vi "te_readVal.vi"(0 "VISA In":refnum<visa-resource-name>, 5 "Hex Address":string="00", 7 "Command":string="01", 11 "Error In":errorcluster) -> (4 "VISA Out":refnum<visa-resource-name>, 6 "Response Dec":dbl, 8 "Response":dbl, 10 "Response Hex":string, 15 "error out":errorcluster)   [LabVIEW 2018]
doc: "The Basic Serial Read and Write example performs a Serial Port Read, a Serial Port Write, or a combination of these actions. The user selects the actions (read or write) on the front panel. If both are selected, the VI will write the data first, read data, and then close the VISA session that is opened to the port. This VI will wait until the specified number of bytes is received at the port. Only the number of bytes specified will be read.\n\nINSTRUCTIONS:\n1) Select the serial resource and configuration parameters (baud rate, data bits, parity, stop bits, flow control).\n2) Select the operations to be performed. \n3) Connect the serial port to your device. If no device is available, perform a loopback test by doing one of the following. Short pins 2 and 3 on a RS-232 cable or short pin 4 to pin 8 and pin 5 to pin 9 on a RS-485/422 cable. \n4) Run the VI to see the data read. (The \"read string\" will match the \"string to write\" if a loopback test was performed.)\n\nNote: The parameters set for the serial port must match the parameters of the connected instrument or device. In this example, the bytes to read parameter specifies the number of bytes that the serial port reads. If there were more bytes at the port than the number specified in bytes to read, those bytes would not be read. Also, if you specify to read more bytes than the number of bytes actually read, you might receive a timeout error message.\n\nOn the block diagram, the Configure Serial Port VI sets the configuration parameters. The front panel displays the controls used to configure the basic parameters, such as baud rate, data bits, and parity. Constants configure the other parameters the user probably does not need set. After the VISA Configure Serial Port VI opens the VISA session and configures the port, the VI passes the VISA resource name to other VIs that perform operations on that VISA resource. The VISA Write function sends a command to the serial device and the VISA Read function returns data based on the command. The VISA Close function then closes the reference to the serial device. It is important to close the reference; otherwise communication through with that port through protocols other than VISA might not be possible."
panel:
  out "ByteCount":i32
  in  "Data":string
  out "Checksum":string
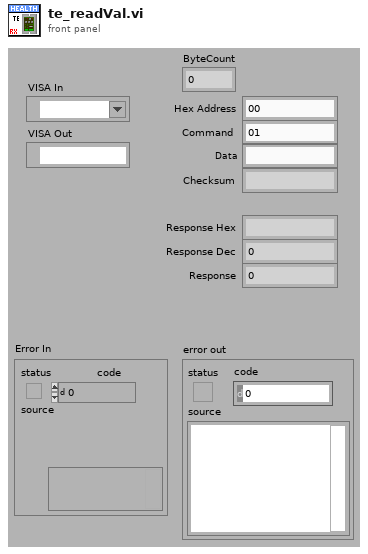
[diagram p1: front panel]
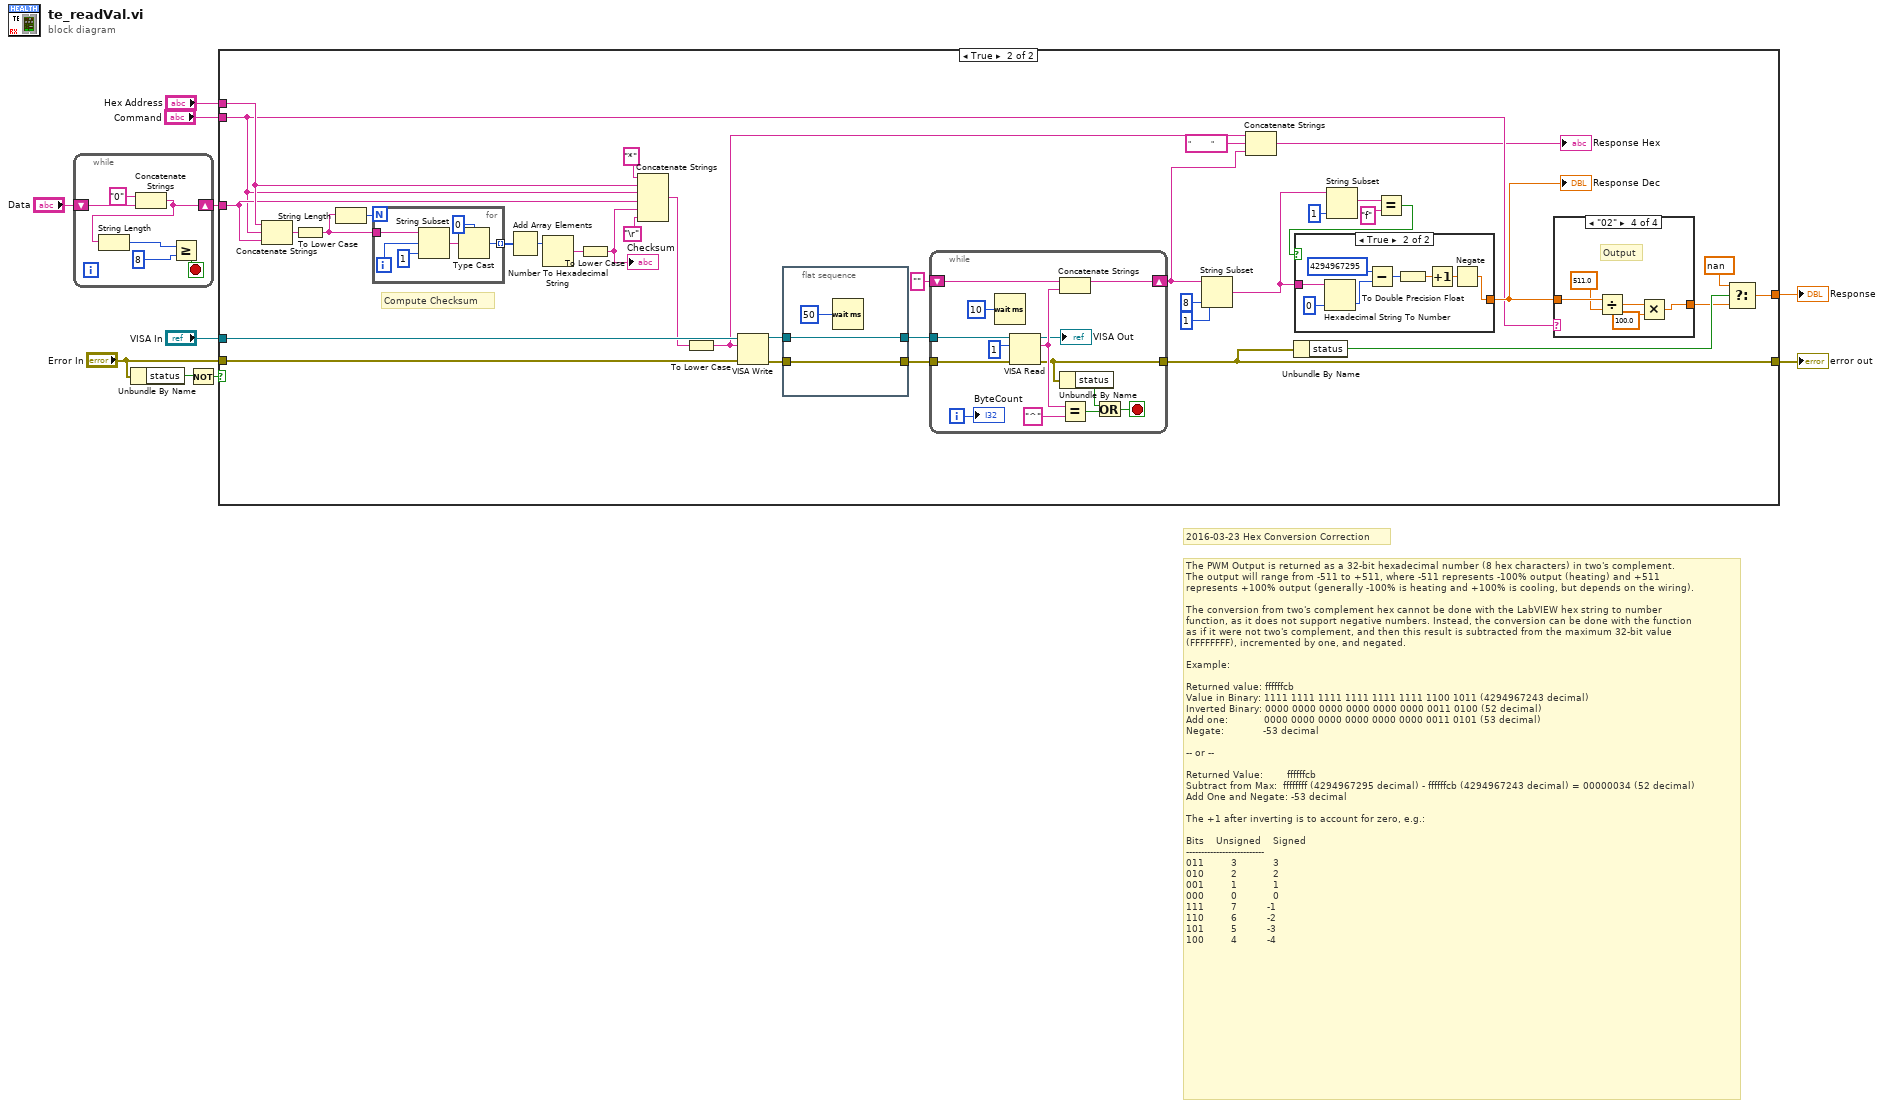
[diagram p0: block diagram]
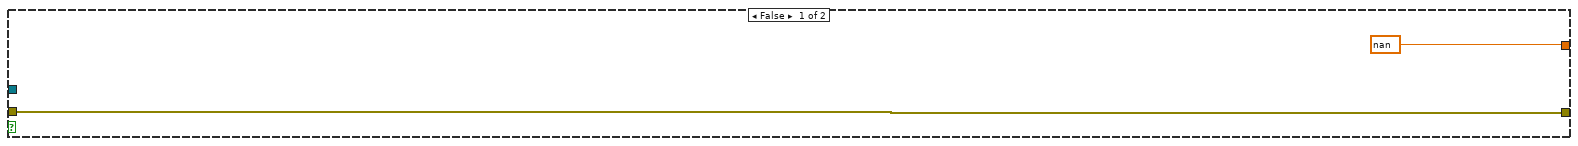
[diagram p2: hidden frame]
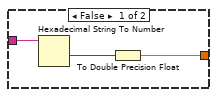
[diagram p3: hidden frame]
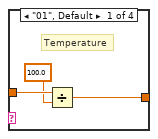
[diagram p4: hidden frame]
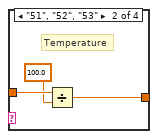
[diagram p5: hidden frame]
diagram:
  # "2016-03-23 Hex Conversion Correction"
  # "The PWM Output is returned as a 32-bit hexadecimal number (8 hex characters) in two's complement.\nThe output will range from -511 to +511, where -511 represents -100% output (heating) and +511\nrepresents +100% output (generally -100% is heating and +100% is cooling, but depends on the wiring).\n\nThe conversion from two's complement hex cannot be done with the LabVIEW hex string to number\nfunction, as it does not support negative numbers. Instead, the conversion can be done with the function\nas if it were not two's complement, and then this result is subtracted from the maximum 32-bit value\n(FFFFFFFF), incremented by one, and negated.\n\nExample:\n\nReturned value: ffffffcb\nValue in Binary: 1111 1111 1111 1111 1111 1111 1100 1011 (4294967243 decimal)\nInverted Binary: 0000 0000 0000 0000 0000 0000 0011 0100 (52 decimal)\nAdd one:            0000 0000 0000 0000 0000 0000 0011 0101 (53 decimal)\nNegate:             -53 decimal\n\n-- or --\n\nReturned Value:        ffffffcb\nSubtract from Max:  ffffffff (4294967295 decimal) - ffffffcb (4294967243 decimal) = 00000034 (52 decimal)\nAdd One and Negate: -53 decimal                \n\nThe +1 after inverting is to account for zero, e.g.:\n\nBits    Unsigned    Signed\n--------------------------\n011         3            3\n010         2            2\n001         1            1\n000         0            0\n111         7          -1\n110         6          -2\n101         5          -3\n100         4          -4"
  n1 = while {
    shift-right: [w14] -> w7
    shift-left: "Data" -> [w16]
    stop <- w11 stop-if-true
    n2 = Concatenate Strings("0" ("string"), w16) -> (w14:string)
    n3 = String Length(string=w14) -> (length=w12:i32)
    n4 = Greater Or Equal?(x=w12, y=8) -> (x >= y?=w11:bool)
  }
  n5 = Unbundle By Name("Error In") -> ("status"=w9:bool)
  n6 = Not(x=w9) -> (.not. x?=w10:bool)
  n7 = case shown="True" w10 {
    tunnel: "VISA In" -> [_ w54]
    tunnel: "Error In" -> [w18 w53]
    tunnel: [w18 w51] -> w8
    tunnel: w7 -> [_ w37]
    tunnel: [nan ("t") w39] -> w6
    tunnel: "Hex Address" -> [_ w38]
    tunnel: "Command" -> [_ w21]
    frame False {
    }
    frame True {
      # "Compute Checksum"
      n8 = Concatenate Strings(w38, w21, w37) -> (w43:string)
      n9 = To Lower Case(string=w43) -> (all lower case string=w45:string)
      n10 = String Length(string=w45) -> (length=w48:i32)
      n11 = for {
        N: w48 -> [_]
        tunnel: w45 -> [w63]
        tunnel: [w59] -> w47 mode=indexing
        i -> [w62]
        n12 = String Subset(string=w63, offset (0)=w62, length (rest)=1 ("length (rest)")) -> (substring=w60:string)
        n13 = Type Cast(type=u8 0, x=w60) -> (*(type *) &x=w59:u8)
      }
      n14 = Add Array Elements(numeric array=w47) -> (sum=w46:u8)
      n15 = Number To Hexadecimal String(2:w46) -> (0:w44:string)  [unwired: 1 in]
      n16 = To Lower Case(string=w44) -> (all lower case string=w42:string)
      "Checksum" <- w42
      n17 = Concatenate Strings("*", w38, w21, w37, w42, "\r") -> (w29:string)
      n18 = To Lower Case(string=w29) -> (all lower case string=w22:string)
      n19 = VISA Write(VISA resource name=w54, write buffer=w22, error in (no error)=w53) -> (VISA resource name out=w27:refnum<visa-resource-name>, error out=w28:errorcluster)  [unwired: 1 out]
      n20 = flat-sequence {
        tunnel: [w57] -> w25
        tunnel: w28 -> [w57]
        tunnel: [w56] -> w26
        tunnel: w27 -> [w56]
        frame #0 {
          n21 = Wait (ms)(milliseconds to wait=u32 50) -> ()  [unwired: 1 out]
        }
      }
      n22 = while {
        tunnel: [w69] -> w51
        tunnel: w26 -> [w71]
        tunnel: w25 -> [w77]
        shift-right: [w75] -> w23
        shift-left: "" ("read buffer") -> [w76]
        i -> [w66]
        stop <- w72 stop-if-true
        n23 = Wait (ms)(milliseconds to wait=u32 10) -> ()  [unwired: 1 out]
        n24 = VISA Read(VISA resource name=w71, byte count=u32 1, error in (no error)=w77) -> (VISA resource name out=→"VISA Out":refnum<visa-resource-name>, read buffer=w74:string, error out=w69:errorcluster)  [unwired: 1 out]
        n25 = Concatenate Strings(w76, w74) -> (w75:string)
        n26 = Unbundle By Name(w69) -> ("status"=w70:bool)
        n27 = Equal?(x=w74, y="^") -> (x = y?=w68:bool)
        n28 = Or(x=w70, y=w68) -> (x .or. y?=w72:bool)
        "ByteCount" <- w66
      }
      n29 = String Subset(string=w23, offset (0)=1, length (rest)=8 ("length (rest)")) -> (substring=w20:string)
      n30 = Concatenate Strings(w22, "          " ("string"), w23) -> (→"Response Hex":string)
      n31 = Unbundle By Name(w51) -> ("status"=w52:bool)
      n32 = String Subset(string=w20, length (rest)=1 ("length (rest)")) -> (substring=w31:string)  [unwired: 1 in]
      n33 = Equal?(x=w31, y="f") -> (x = y?=w33:bool)
      n34 = case shown="True" w33 {
        tunnel: [w80 w84] -> w40
        tunnel: w20 -> [w81 w88]
        frame False {
          n35 = Hexadecimal String To Number(string=w81) -> (number=w79:u32)  [unwired: 2 in, 1 out]
          n36 = To Double Precision Float(number=w79) -> (double precision float=w80:dbl)
        }
        frame True {
          n37 = Hexadecimal String To Number(string=w88, default (0uL)=u32 0 ("default (0 U32)")) -> (number=w86:u32)  [unwired: 1 in, 1 out]
          n38 = Subtract(x=u32 4294967295, y=w86) -> (x-y=w85:u32)
          n39 = To Double Precision Float(number=w85) -> (double precision float=w83:dbl)
          n40 = Increment(x=w83) -> (x+1=w82:dbl)
          n41 = Negate(x=w82) -> (-x=w84:dbl)
        }
      }
      "Response Dec" <- w40
      n42 = case shown="\"02\"" w21 {
        tunnel: w40 -> [w92 w95 w96 w101]
        tunnel: [w90 w93 w96 w97] -> w41
        frame "01", Default {
          # "Temperature"
          n43 = Divide(x=w92, y=100.0) -> (x/y=w90:dbl)
        }
        frame "51", "52", "53" {
          # "Temperature"
          n44 = Divide(x=w95, y=100.0) -> (x/y=w93:dbl)
        }
        frame "05", "44", "45", "46" {
          # "Control Type,\nPolarity"
        }
        frame "02" {
          # "Output"
          n45 = Divide(x=w101, y=511.0) -> (x/y=w99:dbl)
          n46 = Multiply(x=w99, y=100.0) -> (x*y=w97:dbl)
        }
      }
      n47 = Select(t=nan, s=w52, f=w41) -> (s? t:f=w39:dbl)
    }
  }
  "error out" <- w8
  "Response" <- w6
